vi "Main_Test.vi"(8 "Error in":errorcluster, 11 "Queues in":T1) -> (0 "Error out":errorcluster)   [LabVIEW 2019]
uses:
  App/Queue/TypeDef/#TypeDef_App_Queues.ctl
  App/User Interface/TypeDef/#TypeDef_Enum_Buttons.ctl
  App/User Interface/TypeDef/#TypeDef_EventStructureConstant.ctl
  App/User Interface/TypeDef/#TypeDef_Enum_EventStructure.ctl
  App/Queue/TypeDef/#TypeDef_NetworkStream.ctl
  Communication/TypeDef/#TypeDef_FromMRtoPC.ctl
  Communication/TypeDef/#TypeDef_FromPCtoMR.ctl
  Communication/TypeDef/#TypeDef_Command.ctl
  Communication/TypeDef/#TypeDef_ErrorHandler_prop.ctl
  Communication/TypeDef/#TypeDef_PropGraph.ctl
  Communication/TypeDef/#TypeDef_PropertiesToSave.ctl
  <vilib>/addons/database/Connection.llb/Conn ObjectReference.ctl
  TypeDef/#TypeDef_DataToTest.ctl
  TypeDef/#TypeDef_StateAcq.ctl
  TypeDef/#TypeDef_SaveTestData.ctl
  Communication/TypeDef/#TypeDef_SetGet.ctl
  <vilib>/DAQmx/read.llb/DAQmx Read (Analog 1D Wfm NChan NSamp).vi
  <vilib>/DAQmx/create/channels.llb/DAQmx Create Channel (AI-Voltage-Basic).vi
  <vilib>/DAQmx/configure/timing.llb/DAQmx Timing (Sample Clock).vi
  <vilib>/DAQmx/miscellaneous.llb/DAQmx Fill In Error Info.vi
  <vilib>/addons/database/NI_Database_API.lvlib
panel:
  out "Data":waveform(dbl)[](graph)
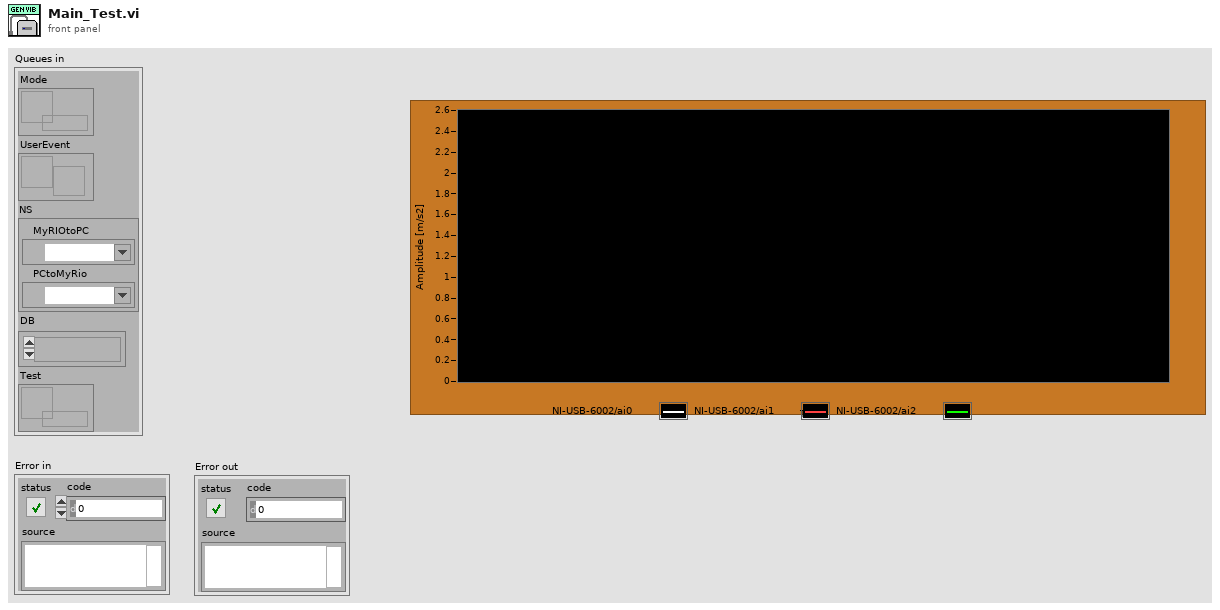
[diagram p1: front panel]
types:
  T1 = typedef "#TypeDef_App_Queues.ctl" = cluster{"Mode":refnum<queue>, "UserEvent":refnum<user-event>, "NS":T2, "DB":T3, "Test":refnum<queue>}
  T2 = typedef "#TypeDef_NetworkStream.ctl" = cluster{"MyRIOtoPC":refnum<k21>, "PCtoMyRio":refnum<k21>}
  T3 = typedef "NI_Database_API.lvlib/Conn ObjectReference.ctl" = refnum<k1>
  T4 = typedef "#TypeDef_StateAcq.ctl" = enum16{"Idle", "Init", "Acq", "End"}
  T5 = typedef "#TypeDef_DataToTest.ctl" = cluster{"FilesPath":path, "Name_Meas":string, "stop":bool, "Command":T6, "Fs":dbl, "Test":bool}
  T6 = typedef "#TypeDef_Command.ctl" = enum16{"Start", "End"}
  T7 = typedef "#TypeDef_SetGet.ctl" = enum16{"Set", "Get"}
  T8 = enum16{"open", "open or create", "create or replace", "create", "open (read-only)"}
  T9 = typedef "#TypeDef_SaveTestData.ctl" = cluster{"data":waveform(dbl)[], "TestData":T5, "Counter":dbl}
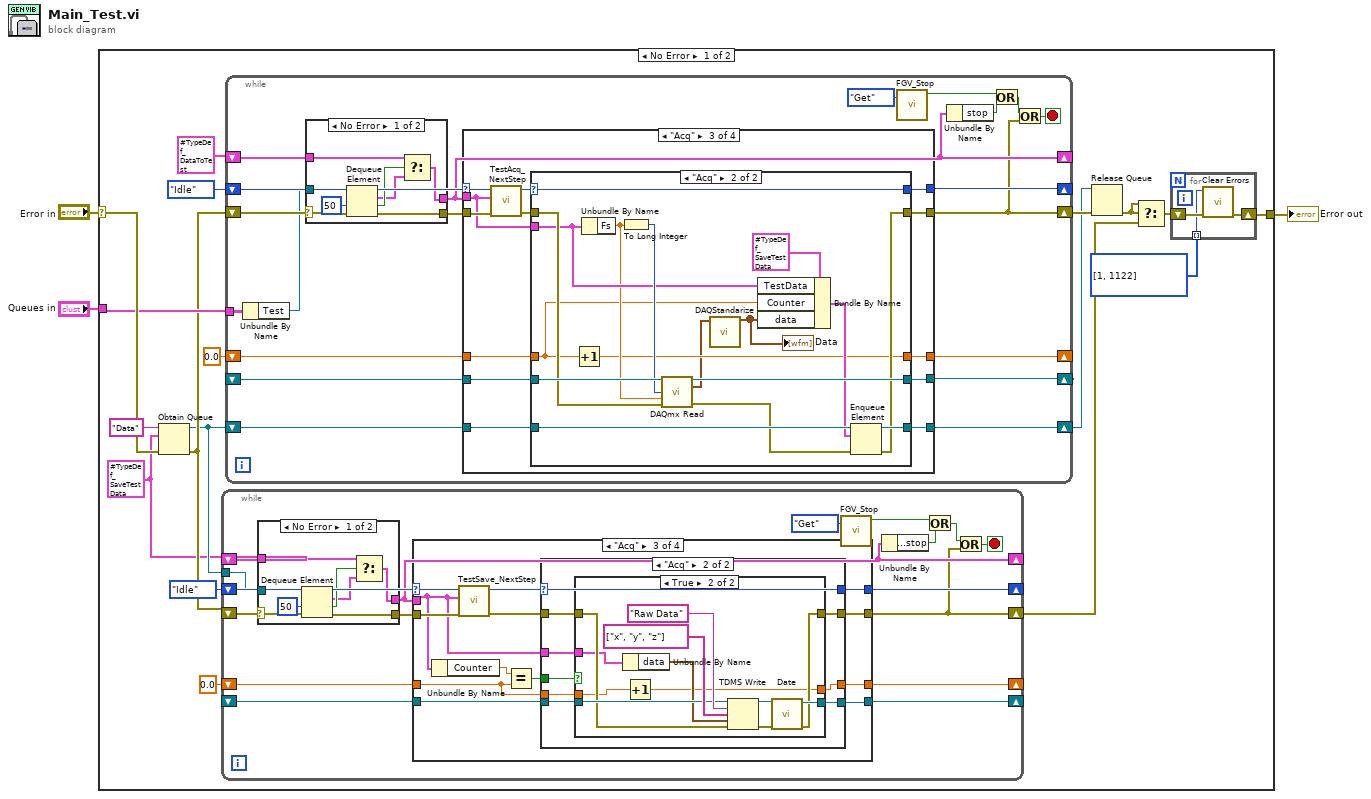
[diagram p0: block diagram]
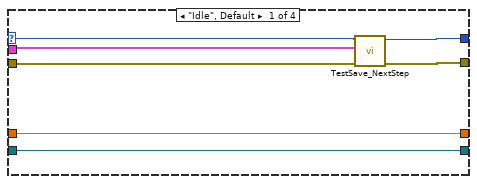
[diagram p3: hidden frame]
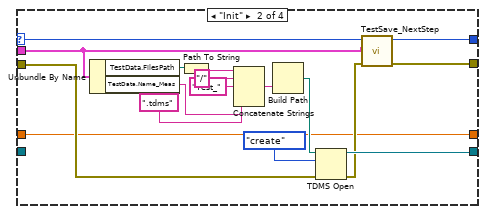
[diagram p4: hidden frame]
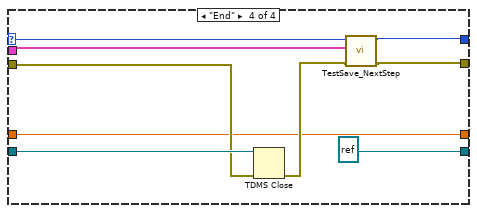
[diagram p7: hidden frame]
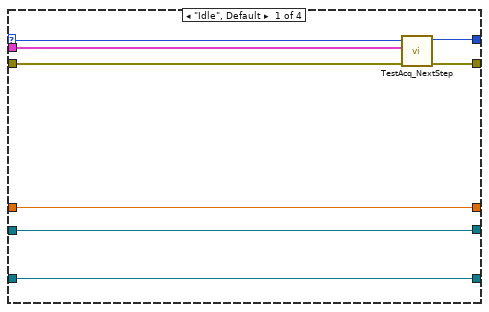
[diagram p9: hidden frame]
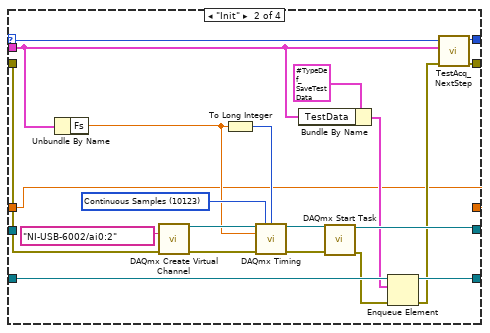
[diagram p10: hidden frame]
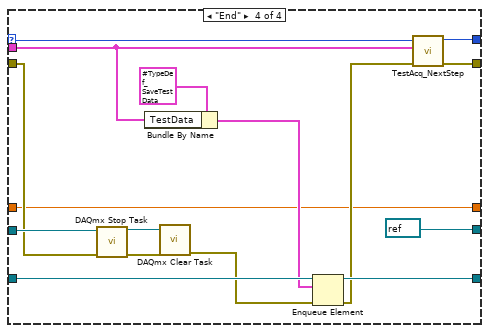
[diagram p12: hidden frame]
diagram:
  n1 = case shown="No Error" "Error in" {
    selector: "Error in" -> [w19 w236]
    tunnel: "Queues in" -> [w18 _]
    tunnel: [w20 w236] -> w2
    frame No Error {
      w6 = T9 {"data"=[], "TestData"={"FilesPath"=path "", "Name_Meas"="", "stop"=FALSE, "Command"=enum."End", "Fs"=1000.0, "Test"=FALSE}, "Counter"=0.0}
      n2 = Obtain Queue(name (unnamed)="Data", element data type=w6, error in (no error)=w19) -> (queue out=w10:refnum<queue>, error out=w15:errorcluster)  [unwired: 2 in, 1 out]
      n3 = while {
        shift-right: [w37] -> _
        shift-left: _ -> [w32]
        shift-right: [w33] -> _
        shift-left: #TypeDef_StateAcq."Idle" -> [w38]
        shift-right: [w30] -> w7
        shift-left: w15 -> [w36]
        shift-right: [w31] -> _
        shift-left: w6 -> [w34]
        tunnel: w10 -> [w24]
        shift-right: [w22] -> _
        shift-left: 0.0 -> [w23]
        stop <- w29 stop-if-true
        n4 = case shown="No Error" w36 {
          selector: w36 -> [w44 w48]
          tunnel: [w45 w48] -> w35
          tunnel: [w43 w47] -> w31
          tunnel: w24 -> [w42 _]
          tunnel: w34 -> [w41 w47]
          frame No Error {
            n5 = Dequeue Element(queue=w42, timeout in ms (-1)=50, error in (no error)=w44) -> (element=w40:T9, timed out?=w46:bool, error out=w45:errorcluster)  [unwired: 1 out]
            n6 = Select(t=w41, s=w46, f=w40) -> (s? t:f=w43:T9)
          }
          frame Error {
          }
        }
        n7 = case shown="\"Acq\"" w38 {
          selector: w38 -> [w52 w59 w82 w119]
          tunnel: [w55 w71 w84 refnum<k34> refnum ("tdms file out")] -> w37
          tunnel: w35 -> [w51 w70 w81 w121]
          tunnel: [w54 w61 w78 w118] -> w33
          tunnel: [w53 w60 w83 w117] -> w30
          tunnel: w31 -> [w50 w57 w77 w115]
          tunnel: w32 -> [w55 _ w85 w122]
          tunnel: w23 -> [w49 w56 w74 w114]
          tunnel: [w49 w56 w73 w114] -> w22
          frame "Idle", Default {
            n8 = call "TestSave_NextStep.vi"("error in"=w51, "SaveTestData"=w50, "Previous Step"=w52) -> ("error out"=w53:errorcluster, "Next Step"=w54:T4)  [unwired: 7 in]
          }
          frame "Init" {
            n9 = Unbundle By Name(w57) -> ("TestData.FilesPath"=w66:path, "TestData.Name_Meas"=w63:string)
            n10 = Path To String(path=w66) -> (string=w69:string)
            n11 = Concatenate Strings(w69, "/" ("string"), "Test_" ("string"), w63, ".tdms" ("string")) -> (w68:string)
            n12 = Build Path(name or relative path=w68) -> (appended path=w65:path)  [unwired: 1 in]
            n13 = TDMS Open(8:w70, 10:T8."create" ("operation (0:open)"), 11:w65) -> (0:w58:errorcluster, 3:w71:refnum<k34>)  [unwired: 4 in]
            n14 = call "TestSave_NextStep.vi"("error in"=w58, "SaveTestData"=w57, "Previous Step"=w59) -> ("error out"=w60:errorcluster, "Next Step"=w61:T4)  [unwired: 7 in]
          }
          frame "Acq" {
            n15 = Unbundle By Name(w77) -> ("Counter"=w76:dbl)
            n16 = call "TestSave_NextStep.vi"("error in"=w81, "SaveTestData"=w77, "Previous Step"=w82) -> ("error out"=w80:errorcluster, "Next Step"=w79:T4)  [unwired: 7 in]
            n17 = Equal?(x=w76, y=w74) -> (x = y?=w75:bool)
            n18 = case shown="\"Acq\"" w79 {
              selector: w79 -> [w89 w93]
              tunnel: w85 -> [w87 w98]
              tunnel: [w87 w97] -> w84
              tunnel: [w88 w96] -> w83
              tunnel: w80 -> [w88 w95]
              tunnel: w77 -> [_ w94]
              tunnel: [w89 w93] -> w78
              tunnel: w75 -> [_ w92]
              tunnel: w74 -> [w86 w91]
              tunnel: [w86 w90] -> w73
              frame "End", Default {
              }
              frame "Acq" {
                n19 = case shown="True" w92 {
                  tunnel: w98 -> [w101 w111]
                  tunnel: [w101 w108] -> w97
                  tunnel: [w99 w106] -> w96
                  tunnel: w95 -> [w99 w105]
                  tunnel: w94 -> [_ w104]
                  tunnel: w91 -> [w100 w103]
                  tunnel: [w100 w102] -> w90
                  frame False {
                  }
                  frame True {
                    n20 = Unbundle By Name(w104) -> ("data"=w107:waveform(dbl)[])
                    n21 = Increment(x=w103) -> (x+1=w102:dbl)
                    n22 = TDMS Write(0:w111, 5:"Raw Data" ("group name in (Untitled)"), 7:string[] ["x", "y", "z"] ("channel name(s) in (Untitled)"), 9:w107, 11:w105) -> (4:w110:refnum<k34>, 15:w109:errorcluster)  [unwired: 1 in, 2 out]
                    n23 = call "Date.vi"("error in"=w109, "Refnum in"=w110) -> ("error out"=w106:errorcluster, "Refnum out"=w108:refnum<k34>)  [unwired: 8 in]
                  }
                }
              }
            }
          }
          frame "End" {
            n24 = TDMS Close(8:w121, 11:w122) -> (0:w116:errorcluster)  [unwired: 1 out]
            n25 = call "TestSave_NextStep.vi"("error in"=w116, "SaveTestData"=w115, "Previous Step"=w119) -> ("error out"=w117:errorcluster, "Next Step"=w118:T4)  [unwired: 7 in]
          }
        }
        n26 = call "FGV_Stop.vi"("Get/Set"=#TypeDef_SetGet."Get") -> ("STOP out"=w27:bool)  [unwired: 10 in]
        n27 = Unbundle By Name(w31) -> ("TestData.stop"=w26:bool)
        n28 = Or(x=w27, y=w26) -> (x .or. y?=w25:bool)
        n29 = Or(x=w25, y=w30) -> (x .or. y?=w29:bool)
      }
      n30 = while {
        shift-right: [w142] -> _
        shift-left: _ -> [w141]
        shift-right: [w134] -> w12
        shift-left: w15 -> [w137]
        shift-right: [w139] -> _
        shift-left: #TypeDef_StateAcq."Idle" -> [w140]
        shift-right: [w135] -> _
        shift-left: T5 {"FilesPath"=path "", "Name_Meas"="", "stop"=FALSE, "Command"=enum."End", "Fs"=1000.0, "Test"=FALSE} -> [w136]
        tunnel: w18 -> [w132]
        shift-right: [w125] -> w9
        shift-left: w10 -> [w126]
        shift-right: [w123] -> _
        shift-left: 0.0 -> [w124]
        stop <- w133 stop-if-true
        n31 = Unbundle By Name(w132) -> ("Test"=w131:refnum<queue>)
        n32 = case shown="No Error" w137 {
          selector: w137 -> [w147 w152]
          tunnel: [w148 w152] -> w138
          tunnel: [w145 w151] -> w135
          tunnel: w131 -> [w144 _]
          tunnel: w136 -> [w143 w151]
          frame No Error {
            n33 = Dequeue Element(queue=w144, timeout in ms (-1)=50, error in (no error)=w147) -> (element=w146:T5, timed out?=w150:bool, error out=w148:errorcluster)  [unwired: 1 out]
            n34 = Select(t=w143, s=w150, f=w146) -> (s? t:f=w145:T5)
          }
          frame Error {
          }
        }
        n35 = case shown="\"Acq\"" w140 {
          selector: w140 -> [w157 w178 w189 w226]
          tunnel: [w160 w181 w193 refnum<k21> refnum ("task out")] -> w142
          tunnel: [w159 w179 w190 w227] -> w134
          tunnel: w138 -> [w156 w176 w188 w218]
          tunnel: w141 -> [w160 _ w194 w232]
          tunnel: [w158 w177 w184 w228] -> w139
          tunnel: w135 -> [w155 w167 w186 w224]
          tunnel: w126 -> [w154 w166 w192 w223]
          tunnel: [w154 w164 w191 w221] -> w125
          tunnel: w124 -> [w153 w161 w183 w217]
          tunnel: [w153 w161 w182 w217] -> w123
          frame "Idle", Default {
            n36 = call "TestAcq_NextStep.vi"("error in"=w156, "TestData"=w155, "Previous Step"=w157) -> ("error out"=w159:errorcluster, "Next Step"=w158:T4)  [unwired: 7 in]
          }
          frame "Init" {
            w171 = 10123 items=["Finite Samples"=10178, "Continuous Samples"=10123, "Hardware Timed Single Point"=12522] ("sample mode")
            n37 = Unbundle By Name(w167) -> ("Fs"=w169:dbl)
            n38 = call-poly <vilib>:"DAQmx Create Virtual Channel.vi"("physical channels"=tag "NI-USB-6002/ai0:2", "error in"=w176) -> ("task out"=w175:refnum<k21>, "error out"=w172:errorcluster)  [unwired: 12 in]
            n39 = To Long Integer(number=w169) -> (32bit integer=w170:i32)
            n40 = call-poly <vilib>:"DAQmx Timing.vi"("task/channels in"=w175, "sample mode"=w171, "samples per channel"=w170, "rate"=w169, "error in"=w172) -> ("task out"=w174:refnum<k21>, "error out"=w173:errorcluster)  [unwired: 9 in]
            n41 = Bundle By Name(cluster=T9 {"data"=[], "TestData"={"FilesPath"=path "", "Name_Meas"="", "stop"=FALSE, "Command"=enum."End", "Fs"=1000.0, "Test"=FALSE}, "Counter"=0.0}, "TestData"=w167) -> (w165:T9)
            n42 = call <vilib>:"DAQmx Start Task.vi"("task/channels in"=w174, "error in"=w173) -> ("task out"=w181:refnum<k21>, "error out"=w163:errorcluster)  [unwired: 12 in]
            n43 = Enqueue Element(queue=w166, element=w165, error in (no error)=w163) -> (queue out=w164:refnum<queue>, error out=w162:errorcluster)  [unwired: 1 in, 1 out]
            n44 = call "TestAcq_NextStep.vi"("error in"=w162, "TestData"=w167, "Previous Step"=w178) -> ("error out"=w179:errorcluster, "Next Step"=w177:T4)  [unwired: 7 in]
          }
          frame "Acq" {
            n45 = call "TestAcq_NextStep.vi"("error in"=w188, "TestData"=w186, "Previous Step"=w189) -> ("error out"=w187:errorcluster, "Next Step"=w185:T4)  [unwired: 7 in]
            n46 = case shown="\"Acq\"" w185 {
              selector: w185 -> [w198 w205]
              tunnel: w194 -> [w196 w216]
              tunnel: [w196 w215] -> w193
              tunnel: w192 -> [w197 w213]
              tunnel: [w197 w210] -> w191
              tunnel: [w199 w208] -> w190
              tunnel: w187 -> [w199 w207]
              tunnel: w186 -> [_ w206]
              tunnel: [w198 w205] -> w184
              tunnel: w183 -> [w195 w203]
              tunnel: [w195 w202] -> w182
              frame "End", Default {
              }
              frame "Acq" {
                n47 = Increment(x=w203) -> (x+1=w202:dbl)
                n48 = Unbundle By Name(w206) -> ("Fs"=w204:dbl)
                n49 = To Long Integer(number=w204) -> (32bit integer=w214:i32)
                n50 = call-poly <vilib>:"DAQmx Read.vi"("task/channels in"=w216, "number of samples per channel"=w214, "timeout"=w204, "error in"=w207) -> ("task out"=w215:refnum<k21>, "data"=w201:waveform(dbl)[], "error out"=w211:errorcluster)  [unwired: 9 in]
                n51 = call "DAQStandarize.vi"("Data in"=w201) -> ("Data out"=w200:waveform(dbl)[])  [unwired: 10 in]
                "Data" <- w200
                n52 = Bundle By Name(cluster=T9 {"data"=[], "TestData"={"FilesPath"=path "", "Name_Meas"="", "stop"=FALSE, "Command"=enum."End", "Fs"=1000.0, "Test"=FALSE}, "Counter"=0.0}, "TestData"=w206, "Counter"=w203, "data"=w200) -> (w212:T9)
                n53 = Enqueue Element(queue=w213, element=w212, error in (no error)=w211) -> (queue out=w210:refnum<queue>, error out=w208:errorcluster)  [unwired: 1 in, 1 out]
              }
            }
          }
          frame "End" {
            n54 = call <vilib>:"DAQmx Stop Task.vi"("task/channels in"=w232, "error in"=w218) -> ("task out"=w231:refnum<k21>, "error out"=w230:errorcluster)  [unwired: 12 in]
            n55 = Bundle By Name(cluster=T9 {"data"=[], "TestData"={"FilesPath"=path "", "Name_Meas"="", "stop"=FALSE, "Command"=enum."End", "Fs"=1000.0, "Test"=FALSE}, "Counter"=0.0}, "TestData"=w224) -> (w222:T9)
            n56 = call <vilib>:"DAQmx Clear Task.vi"("task in"=w231, "error in"=w230) -> ("error out"=w220:errorcluster)  [unwired: 13 in]
            n57 = Enqueue Element(queue=w223, element=w222, error in (no error)=w220) -> (queue out=w221:refnum<queue>, error out=w219:errorcluster)  [unwired: 1 in, 1 out]
            n58 = call "TestAcq_NextStep.vi"("error in"=w219, "TestData"=w224, "Previous Step"=w226) -> ("error out"=w227:errorcluster, "Next Step"=w228:T4)  [unwired: 7 in]
          }
        }
        n59 = call "FGV_Stop.vi"("Get/Set"=#TypeDef_SetGet."Get") -> ("STOP out"=w129:bool)  [unwired: 10 in]
        n60 = Unbundle By Name(w135) -> ("stop"=w128:bool)
        n61 = Or(x=w129, y=w128) -> (x .or. y?=w127:bool)
        n62 = Or(x=w127, y=w134) -> (x .or. y?=w133:bool)
      }
      n63 = Release Queue(queue=w9, error in (no error)=w12) -> (error out=w8:errorcluster)  [unwired: 1 in, 2 out]
      n64 = Select(t=w8, s=w8, f=w7) -> (s? t:f=w17:errorcluster)
      n65 = for {
        shift-right: [w234] -> w20
        shift-left: w17 -> [w235]
        tunnel: i32[] [1, 1122] -> [w233] mode=indexing
        n66 = call <vilib>:"Clear Errors.vi"("error in (no error)"=w235, "specific error code to clear (0: all)"=w233) -> ("error out"=w234:errorcluster)  [unwired: 4 in, 1 out]
      }
    }
    frame Error {
    }
  }
  "Error out" <- w2
